vi "AOL Z Cal-Process window.vi"(8 "error in (no error)":errorcluster) -> (0 "error out":errorcluster, 1 "Cancelled (Left button pressed)":bool, 3 "Timed out while waiting for acknowledgement":bool)   [LabVIEW 2020]
doc: "Use this template to create a dialog box with event handling."
uses:
  Typedefs/AOL Z cal process refs.ctl
  <vilib>/Utility/miscctls.llb/LVPointTypeDef.ctl
  Typedefs/Top level VI states.ctl
  Typedefs/Functional global standard states.ctl
  Globals/gl_Calibration globals.vi
  Global Variables/General Globals.vi
panel:
  out "Progress bar":u8(slide) scale=0.0..100.0
  out "Next (ind)":bool
  in  "Delay":u32=1000
  out "Cancelled/Aborted":bool
  out "Exit":bool
  out "Abort (ind)":bool
  out "Cal":sgl[][](array[numeric])
  out "Display message":string
  in  "Cancel":bool
  in  "Next":bool
  in  "Message string":string
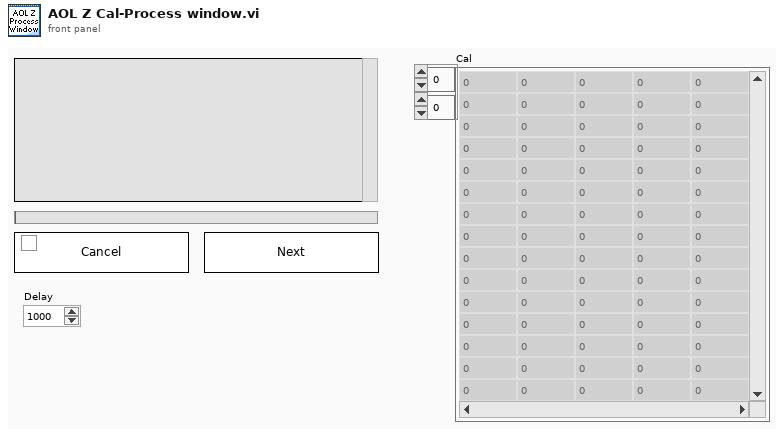
[diagram p1: front panel]
types:
  T1 = typedef "AOL Z cal process refs.ctl" = cluster{"This VI":refnum<vi>, "Abort (ind)":refnum<vi>, "Next (ind)":refnum<vi>, "Cancel":refnum<vi>, "Next":refnum<vi>, "Message":refnum<vi>, "Progress":refnum<vi>}
  T2 = typedef "LVPointTypeDef.ctl" = cluster{"Horizontal":i16, "Vertical":i16}
  T3 = typedef "Cal points.ctl" = enum16{"5-points calibration (crude)", "11-points calibration", "21-points calibration", "41-points calibration"}
  T4 = typedef "FOV values cluster.ctl" = cluster{"Norm value":sgl, "FOV text":string, "FOV value":i32, "All FOV values":i32[], "All norm FOV values":sgl[], "All FOV value strings":string[], "Strings And Values []":T5}
  T5 = typedef "LVStringsAndValuesArrayTypeDef_SGL.ctl" = cluster{"String":string, "Value":sgl}[]
  T6 = typedef "Functional global standard states.ctl" = enum16{"Initialise", "Read", "Write", "Load", "Save", "Clear"}
  T7 = typedef "Top level VI states.ctl" = enum16{"None", "Initialise UI", "<STACK PROTOCOL STATES>", "AOL Zstack-START", "AOL Zstack-STOP", "Motor Zstack-START", "Motor Zstack-STOP", "Parameter Sweep-START", "Parameter Sweep-STOP", "<ACQUISITION PROTOCOL STATES> ", "Functional Acquisition-START", "Functional Acquisition-STOP", "Single Plane Acquisition-START", "Single Plane Acquisition-STOP", "Volume Acquisition-START", "Volume Acquisition-STOP", "<LIVE IMAGING PROTOCOL STATES>", "Live Imaging-START", "Live Imaging-STOP", "Live Plane Imaging-START", "Live Plane Imaging-STOP", "Live Volume Imaging-START", "Live Volume Imaging-STOP", "<MOVEMENT CORRECTION PROTOCOL STATES>", "EXIT"}
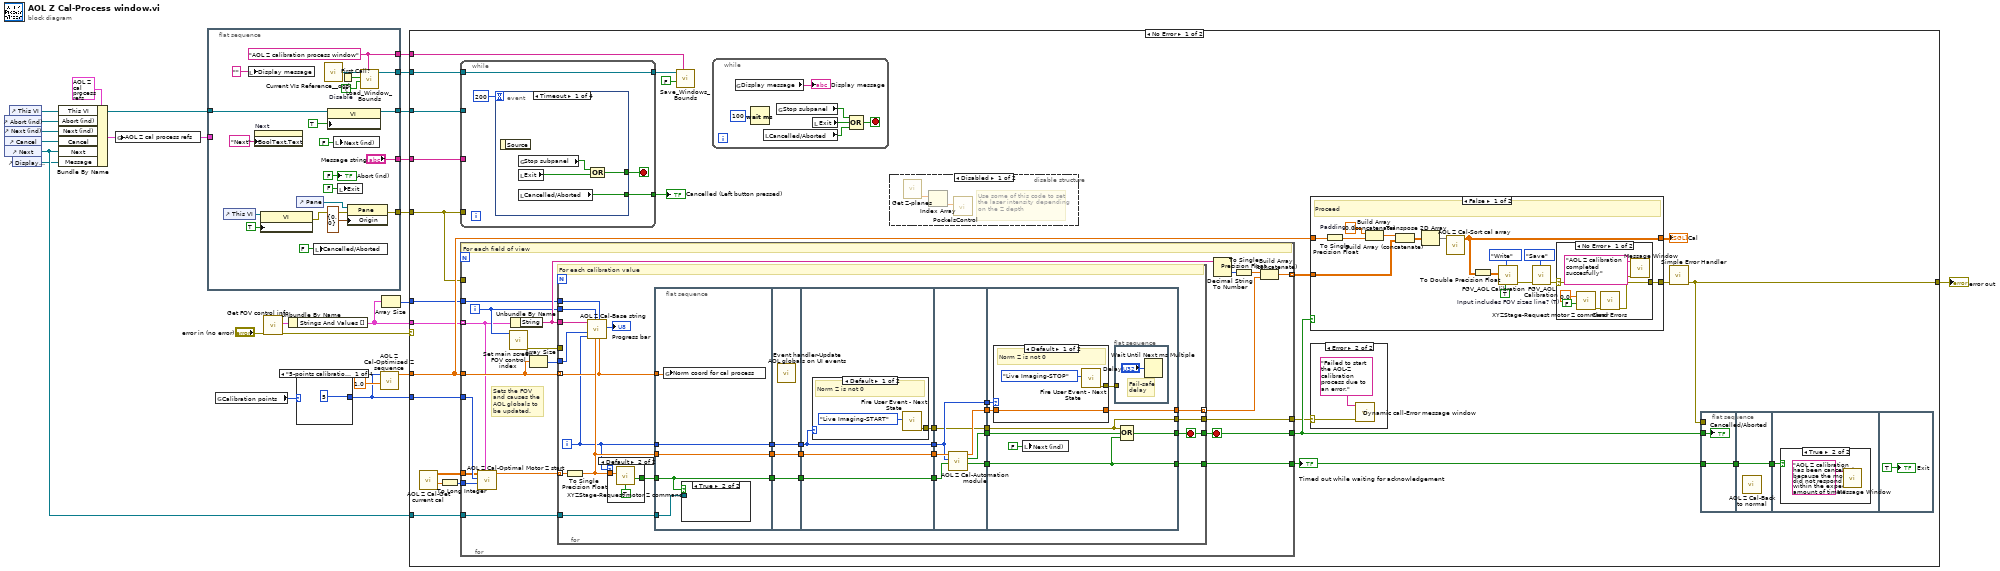
[diagram p0: block diagram]
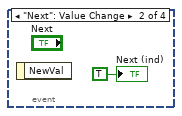
[diagram p7: hidden frame]
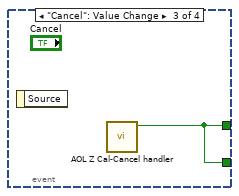
[diagram p8: hidden frame]
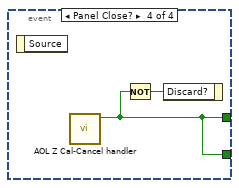
[diagram p9: hidden frame]
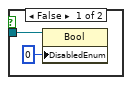
[diagram p11: hidden frame]
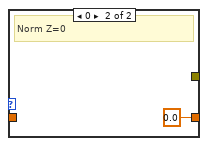
[diagram p13: hidden frame]
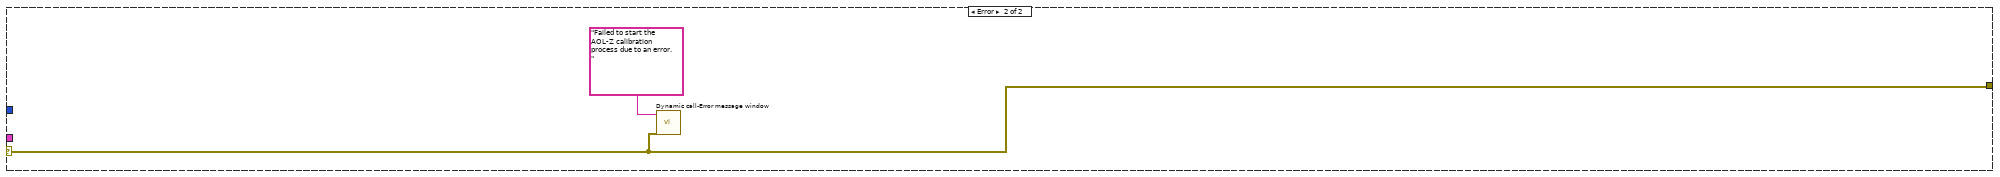
[diagram p14: hidden frame]
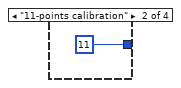
[diagram p15: hidden frame]
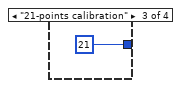
[diagram p16: hidden frame]
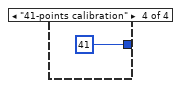
[diagram p17: hidden frame]
diagram:
  n1 = control-ref of="Abort (ind)"() -> (w14:refnum<vi>)
  n2 = control-ref of="Next (ind)"() -> (w13:refnum<vi>)
  n3 = control-ref of="Cancel"() -> (w12:refnum<vi>)
  n4 = control-ref of="Next"() -> (w11:refnum<vi>)
  n5 = control-ref of="This VI"() -> (w10:refnum<vi>)
  n6 = control-ref of="Display message"() -> (w9:refnum<vi>)
  n7 = Bundle By Name(cluster=T1 {"This VI"=refnum, "Abort (ind)"=refnum, "Next (ind)"=refnum, "Cancel"=refnum, "Next"=refnum, "Message"=refnum, "Progress"=refnum} ("AOL Z cal wizard refs"), "This VI"=w10, "Abort (ind)"=w14, "Next (ind)"=w13, "Cancel"=w12, "Next"=w11, "Message"=w9) -> (w8:T1)
  n8 = global write "gl_Calibration globals.vi" "AOL Z cal process refs"(w8) -> ()
  n9 = flat-sequence {
    tunnel: ["Message string"] -> w23
    tunnel: [w42] -> w22
    tunnel: [w40] -> w17
    tunnel: [w35] -> w21
    tunnel: [w34] -> w20
    tunnel: w8 -> [_]
    tunnel: w10 -> [w24]
    frame #0 {
      w36 = FALSE  # Disable
      w35 = "AOL Z calibration process window" ("Window Name (i.e. Key)")
      n10 = control-ref of="This VI"() -> (w26:refnum<vi>)
      n11 = local write "Display message"("" ("Status")) -> ()
      n12 = property on="Next" class="Bool"("BoolText.Text"="Next" ("Boolean Text.Text")) -> ()  [unwired: 2 in, 2 out]
      n13 = property on="Property Node" class="VI"(reference=w26, "Front Panel.IsFrontmost"=TRUE ("Front Panel Window:Is Frontmost")) -> (error out=w25:errorcluster)  [unwired: 1 in, 1 out]
      n14 = control-ref of="Pane"() -> (w39:refnum<vi>)
      n15 = local write "Cancelled/Aborted"(FALSE ("Completed")) -> ()
      n16 = call <userlib>:"Current VIs Reference__ogtk.vi"() -> ("Current VI's reference"=w38:refnum<vi>)  [unwired: 5 in]
      n17 = property on="Property Node" class="VI"(reference=w24, "Front Panel.IsFrontmost"=TRUE ("Front Panel Window:Is Frontmost")) -> (reference out=w42:refnum<vi>)  [unwired: 1 in, 1 out]
      n18 = local write "Next (ind)"(FALSE ("Next (ind)")) -> ()
      n19 = local write "Exit"(FALSE ("Finished")) -> ()
      n20 = First Call?() -> (First Call?: T/F=w37:bool)
      n21 = property class="Pane"(reference=w39, error in=w25, "Origin"=T2 {"Horizontal"=0, "Vertical"=0}) -> (error out=w40:errorcluster)  [unwired: 1 out]
      n22 = call "Load_Window_Bounds.vi"("Window Name (i.e. Key)"=w35, "Disable"=w36, "First Call"=w37, "Window VI's Ref"=w38) -> ("reference out"=w34:refnum<vi>)  [unwired: 4 in, 3 out]
      "Abort (ind)" <- FALSE ("Cancel ind")
    }
  }
  n23 = global read "gl_Calibration globals.vi" "Calibration points"() -> (w5:T3)
  n24 = call "Get FOV control info.vi"("error in (no error)"="error in (no error)") -> ("error out"=w3:errorcluster, "FOV values cluster"=w19:T4)  [unwired: 7 in, 2 out]
  n25 = Unbundle By Name(w19) -> ("Strings And Values []"=w16:T5)
  n26 = case shown="\"5-points calibration (crude)\", Default" w5 {
    tunnel: [5 ("Calibration points") 11 ("Calibration points") 21 ("Calibration points") 41 ("Calibration points")] -> w4
    frame "5-points calibration (crude)", Default {
    }
    frame "11-points calibration" {
    }
    frame "21-points calibration" {
    }
    frame "41-points calibration" {
    }
  }
  n27 = call "AOL Z Cal-Optimised Z sequence.vi"("Max positive value"=1.0, "Calibration points"=w4) -> ("Calibration's optimised norm Z sequence"=w18:dbl[])  [unwired: 8 in, 1 out]
  n28 = Array Size(array=w16) -> (size(s)=w7:i32)
  n29 = case shown="No Error" w3 {
    selector: w3 -> [_ w213]
    tunnel: w23 -> [w71 _]
    tunnel: w22 -> [w70 _]
    tunnel: w21 -> [w68 _]
    tunnel: w20 -> [w66 _]
    tunnel: w18 -> [w64 _]
    tunnel: w17 -> [w61 _]
    tunnel: w16 -> [w59 _]
    tunnel: w11 -> [w55 _]
    tunnel: w7 -> [w52 _]
    tunnel: w4 -> [w51 _]
    tunnel: [w50 w213] -> w1
    frame No Error {
      n30 = call "AOL Z Cal-Get current cal.vi"() -> ("FOVs"=w57:dbl[], "Previous cal"=w58:dbl[][])  [unwired: 10 in]
      n31 = To Long Integer(number=w57) -> (32bit integer=w56:i32[])
      n32 = while {
        tunnel: w71 -> [_]
        tunnel: w61 -> [_]
        tunnel: w70 -> [_]
        tunnel: [w113] -> w69
        tunnel: w66 -> [w112]
        tunnel: [w112] -> w65
        stop <- w115 stop-if-true
        n33 = event shown="[0] Timeout" {
          selector: _ -> [_ _ _ _]
          dyn-events: _ -> [_ _ _ _]
          timeout: 200 -> [_ _ _ _]
          tunnel: [w118 _ w121 w123] -> w115
          tunnel: [w116 _ w121 w123] -> w113
          event Timeout {
            n34 = event-data() -> ()  [unwired: 1 in, 1 out]
            n35 = global read "General Globals.vi" "Stop subpanel"() -> (w117:bool)
            n36 = local read "Exit"() -> (w119:bool)
            n37 = local read "Cancelled/Aborted"() -> (w116:bool)
            n38 = Compound Arithmetic op=OR(w117, w119) -> (w118:bool)
          }
          event "Next": Value Change {
            n39 = event-data() -> ()  [unwired: 1 in, 1 out]
            "Next (ind)" <- TRUE ("Next (ind)")
          }
          event "Cancel": Value Change {
            n40 = event-data() -> ()  [unwired: 1 in, 1 out]
            n41 = call "AOL Z Cal-Cancel handler.vi"() -> ("Stop?"=w121:bool)  [unwired: 11 in]
          }
          event Panel Close? {
            n42 = event-data() -> ()  [unwired: 1 in, 1 out]
            n43 = call "AOL Z Cal-Cancel handler.vi"() -> ("Stop?"=w123:bool)  [unwired: 11 in]
            n44 = Not(x=w123) -> (.not. x?=w122:bool)
            n45 = event-data("Discard?"=w122) -> ()  [unwired: 1 in, 1 out]
          }
        }
      }
      "Cancelled (Left button pressed)" <- w69
      n46 = for {
        tunnel: w64 -> [w135]
        tunnel: w59 -> [w125] mode=indexing
        tunnel: w55 -> [w141]
        tunnel: [w137] -> w63 mode=indexing
        tunnel: [w136] -> w53
        tunnel: w61 -> [_]
        tunnel: w51 -> [w131]
        tunnel: [w134] -> w54
        tunnel: w58 -> [w129]
        tunnel: w56 -> [w132]
        tunnel: w52 -> [w128]
        tunnel: [w124] -> w49
        i -> [w127]
        stop <- w136 stop-if-true
        # "Sets the FOV and causes the AOL globals to be updated."
        # "For each field of view"
        n47 = call "AOL Z Cal-Optimal Motor Z start.vi"("FOV info"=w125, "FOVs"=w132, "Desired # cal points"=w131, "Current Cal (no Norm Z column)"=w129) -> ("Optimal motor Z start positions"=w130:dbl[])  [unwired: 7 in]
        n48 = call "Set main screen FOV control index.vi"("FOV control index"=w127) -> ("error out"=w142:errorcluster)  [unwired: 10 in]
        n49 = Unbundle By Name(w125) -> ("String"=w133:string)
        n50 = Array Size(array=w135) -> (size(s)=w126:i32)
        n51 = for {
          tunnel: w135 -> [w151] mode=indexing
          tunnel: w142 -> [_]
          tunnel: w133 -> [w156]
          tunnel: w141 -> [w150]
          tunnel: [w172] -> w138 mode=indexing
          tunnel: [w170] -> w136
          tunnel: w126 -> [w169]
          tunnel: w130 -> [w165] mode=indexing
          tunnel: [w166] -> w134
          tunnel: w128 -> [w148]
          tunnel: w127 -> [w147]
          tunnel: [w143] -> w124
          i -> [w149]
          stop <- w170 stop-if-true
          # "For each calibration value"
          n52 = To Single Precision Float(number=w165) -> (single precision float=w155:sgl)
          n53 = call "AOL Z Cal-Base string.vi"("Norm coord for cal process"=w151, "Number of FOVs"=w148, "Initial motor Z"=w155, "Index of current FOV"=w147, "Index of current Cal point"=w149, "Number of Cal points (per FOV)"=w169, "FOV (string)"=w156) -> ("Progress %"=→"Progress bar":u8)  [unwired: 4 in]
          n54 = case shown="Default" w149 {
            tunnel: w155 -> [_ w174]
            tunnel: [_ w173] -> w160
            frame 0 {
            }
            frame Default {
              n55 = call "XYZStage-Request motor Z command.vi"("Wait for acknowledge?"=TRUE, "Motor Z"=w174) -> ("Timed out while waiting for acknowledgement"=w173:bool)  [unwired: 7 in, 2 out]
            }
          }
          n56 = flat-sequence {
            tunnel: w155 -> [w179]
            tunnel: w149 -> [w180]
            tunnel: w160 -> [w176]
            tunnel: [w176] -> w154
            tunnel: [w180] -> w153
            tunnel: [w179] -> w152
            tunnel: w151 -> [w178]
            tunnel: w150 -> [w177]
            tunnel: [w185] -> w163
            tunnel: [w184] -> w161
            tunnel: [w183] -> w158
            tunnel: w154 -> [w185]
            tunnel: w153 -> [w184]
            tunnel: w152 -> [w183]
            tunnel: [w187] -> w168
            tunnel: [w188] -> w164
            tunnel: w163 -> [w187]
            tunnel: w161 -> [w188]
            tunnel: [w189] -> w159
            tunnel: w158 -> [w189]
            tunnel: [w186] -> w144
            tunnel: [w195] -> w171
            tunnel: w168 -> [w198]
            tunnel: [w196] -> w167
            tunnel: w164 -> [w193]
            tunnel: [w193] -> w162
            tunnel: w159 -> [w197]
            tunnel: [w194] -> w157
            tunnel: [w192] -> w145
            tunnel: w144 -> [w192]
            tunnel: w171 -> [w205]
            tunnel: w167 -> [w204]
            tunnel: w162 -> [w206]
            tunnel: [w201] -> w172
            tunnel: [w204] -> w166
            tunnel: [w203] -> w170
            tunnel: w157 -> [w200]
            tunnel: w145 -> [w199]
            tunnel: [w199] -> w143
            frame #0 {
              n57 = global write "gl_Calibration globals.vi" "Norm coord for cal process"(w178) -> ()
              n58 = case shown="True" w176 {
                tunnel: w177 -> [w182 _]
                frame False {
                  n59 = property class="Bool"(reference=w182, "DisabledEnum"=0) -> ()  [unwired: 1 in, 2 out]
                }
                frame True {
                }
              }
            }
            frame #1 {
              n60 = call "Event handler-Update AOL globals on UI events.vi"() -> ()  [unwired: 11 in, 1 out]
            }
            frame #2 {
              n61 = case shown="Default" w188 {
                tunnel: [w190 _] -> w186
                frame Default {
                  # "Norm Z is not 0"
                  n62 = call "Fire User Event - Next State.vi"("\"UI Handler loop\" case to execute"=Top_level_VI_states."Live Imaging-START" ("\"UI Handler loop\" case to execute")) -> ("Error Out"=w190:errorcluster)  [unwired: 10 in]
                }
                frame 0 {
                  # "Norm Z=0"
                }
              }
            }
            frame #3 {
              n63 = call "AOL Z Cal-Automation module.vi"("Timed out while waiting for acknowledgement in"=w198, "FOR loop index"=w193, "Initial motor position (um)"=w197) -> ("Motor timed out or errored out"=w196:bool, "Cancelled"=w195:bool, "Measured cal value"=w194:sgl)  [unwired: 6 in]
            }
            frame #4 {
              n64 = case shown="Default" w206 {
                tunnel: [w210 _] -> w202
                tunnel: [w209 sgl 0.0 ("Z")] -> w201
                tunnel: w200 -> [w209 _]
                frame Default {
                  # "Norm Z is not 0"
                  n65 = call "Fire User Event - Next State.vi"("\"UI Handler loop\" case to execute"=Top_level_VI_states."Live Imaging-STOP" ("\"UI Handler loop\" case to execute")) -> ("Error Out"=w210:errorcluster)  [unwired: 10 in]
                }
                frame 0 {
                  # "Norm Z=0"
                }
              }
              n66 = local write "Next (ind)"(FALSE ("Next (ind)")) -> ()
              n67 = flat-sequence {
                tunnel: w202 -> [_]
                frame #0 {
                  # "Fail-safe delay"
                  n68 = Wait Until Next ms Multiple(millisecond multiple="Delay") -> ()  [unwired: 1 out]
                }
              }
              n69 = Compound Arithmetic op=OR(w199, w205, w204) -> (w203:bool)
            }
          }
        }
        n70 = Decimal String To Number(string=w133) -> (number=w140:i32)  [unwired: 2 in, 1 out]
        n71 = To Single Precision Float(number=w140) -> (single precision float=w139:sgl)
        n72 = Build Array (concatenate)(w139, w138) -> (w137:sgl[])
      }
      "Timed out while waiting for acknowledgement" <- w54
      n73 = call "Save_Windows_Bounds.vi"("Window Name (i.e. Key)"=w68, "Front Panel Window:Open"=FALSE, "Window VI's Ref"=w65) -> ()  [unwired: 8 in, 1 out]
      n74 = while {
        stop <- w79 stop-if-true
        n75 = global read "gl_Calibration globals.vi" "Display message"() -> (→"Display message":string)
        n76 = Wait (ms)(milliseconds to wait=u32 100) -> ()  [unwired: 1 out]
        n77 = local read "Cancelled/Aborted"() -> (w76:bool)
        n78 = global read "General Globals.vi" "Stop subpanel"() -> (w81:bool)
        n79 = local read "Exit"() -> (w80:bool)
        n80 = Compound Arithmetic op=OR(w81, w80, w76) -> (w79:bool)
      }
      n81 = disable-structure shown="Disabled" {
        frame Disabled {
          # "Use some of this code to set the laser intensity depending on the Z depth"
          n82 = call "Get Z-planes.vi"() -> ("Pockels vs. Z (Laser power %)"=w89:dbl[])  [unwired: 7 in, 4 out]
          n83 = Index Array(array=w89) -> (element=w88:dbl)  [unwired: 1 in]
          n84 = call "PockelsControl.vi"("Laser Power (%)"=w88) -> ()  [unwired: 10 in, 1 out]
        }
        frame Enabled {
        }
      }
      n85 = case shown="False" w53 {
        tunnel: w64 -> [w103 _]
        tunnel: w63 -> [w101 _]
        tunnel: [w94 _] -> w62
        tunnel: [w90 _] -> w60
        frame False {
          w92 = TRUE  # Input includes FOV sizes line? (T)
          w104 = sgl 0.0  # Padding
          # "Proceed"
          n86 = To Single Precision Float(number=w103) -> (single precision float=w100:sgl[])
          n87 = Build Array (concatenate)(w104, w100) -> (w102:sgl[])
          n88 = Build Array (concatenate)(w102, w101) -> (w99:sgl[][])
          n89 = Transpose 2D Array(2D array=w99) -> (transposed array=w98:sgl[][])
          n90 = call "AOL Z Cal-Sort cal array.vi"("Unsorted cal"=w98) -> ("Sorted cal"=w94:sgl[][])  [unwired: 10 in]
          n91 = To Double Precision Float(number=w94) -> (double precision float=w93:dbl[][])
          n92 = call "FGV_AOL Calibration.vi"("Input includes FOV sizes line? (T)"=w92, "Function"=Functional_global_standard_states."Write", "Calibration Data in"=w93) -> ("error out"=w96:errorcluster)  [unwired: 6 in, 2 out]
          n93 = call "FGV_AOL Calibration.vi"("error in (no error)"=w96, "Function"=Functional_global_standard_states."Save") -> ("error out"=w91:errorcluster)  [unwired: 7 in, 2 out]
          n94 = case shown="No Error" w91 {
            selector: w91 -> [w110 w111]
            tunnel: [w110 w111] -> w90
            frame No Error {
              n95 = call "XYZStage-Request motor Z command.vi"("Wait for acknowledge?"=FALSE, "Motor Z"=sgl 0.0) -> ("error out"=w108:errorcluster)  [unwired: 7 in, 2 out]
              n96 = call <vilib>:"Clear Errors.vi"("error in (no error)"=w108) -> ("error out"=w106:errorcluster)  [unwired: 5 in, 1 out]
              n97 = call "Message Window.vi"("error in (no error)"=w106, "Message string"="AOL Z calibration completed succesfully") -> ()  [unwired: 9 in, 1 out]
            }
            frame Error {
            }
          }
        }
        frame True {
          # "Cancelled/Aborted"
        }
      }
      "Cal" <- w62
      n98 = case shown="Error" w49 {
        selector: w49 -> [_ w75]
        frame No Error {
        }
        frame Error {
          n99 = call "Dynamic call-Error message window.vi"("error in (no error)"=w75, "Error Message"="Failed to start the AOL-Z calibration process due to an error.") -> ()  [unwired: 9 in, 1 out]
        }
      }
      n100 = call <vilib>:"Simple Error Handler.vi"("error in (no error)"=w60) -> ("error out"=w50:errorcluster)  [unwired: 4 in, 4 out]
      n101 = flat-sequence {
        tunnel: w54 -> [w83]
        tunnel: [w83] -> w73
        tunnel: w53 -> [w82]
        tunnel: w50 -> [_]
        tunnel: [w84] -> w72
        tunnel: w73 -> [w84]
        tunnel: w72 -> [w85]
        frame #0 {
          "Cancelled/Aborted" <- w82
        }
        frame #1 {
          n102 = call "AOL Z Cal-Back to normal.vi"() -> ()  [unwired: 12 in]
        }
        frame #2 {
          n103 = case shown="True" w85 {
            frame False {
            }
            frame True {
              n104 = call "Message Window.vi"("Message string"="AOL Z calibration has been cancelled because the motor did not respond within the expected amount of time.") -> ()  [unwired: 10 in, 1 out]
            }
          }
        }
        frame #3 {
          "Exit" <- TRUE ("Finished")
        }
      }
    }
    frame Error {
      n105 = call "Dynamic call-Error message window.vi"("error in (no error)"=w213, "Error Message"="Failed to start the AOL-Z calibration process due to an error.") -> ()  [unwired: 9 in, 1 out]
    }
  }
  "error out" <- w1
